vi "Write setSpectTempSetpoint.vi"(8 "error in (no error)":errorcluster, 10 "command_setSpectTempSetpoint":T1, 11 "setSpectTempSetpoint in":refnum<class "setSpectTempSetpoint.lvclass">) -> (0 "error out":errorcluster, 3 "setSpectTempSetpoint out":refnum<class "setSpectTempSetpoint.lvclass">)   [LabVIEW 2016, in "Commands.lvlib" / "setSpectTempSetpoint.lvclass"]
uses:
  setSpectTempSetpoint.lvclass
  ts_sallv_sedspectrometer/DataTypes/command_setSpectTempSetpoint.ctl
  setSpectTempSetpoint.lvclass/setSpectTempSetpoint.ctl
  ts_sallv_sedspectrometer/SALLV_sedSpectrometer.lvlib
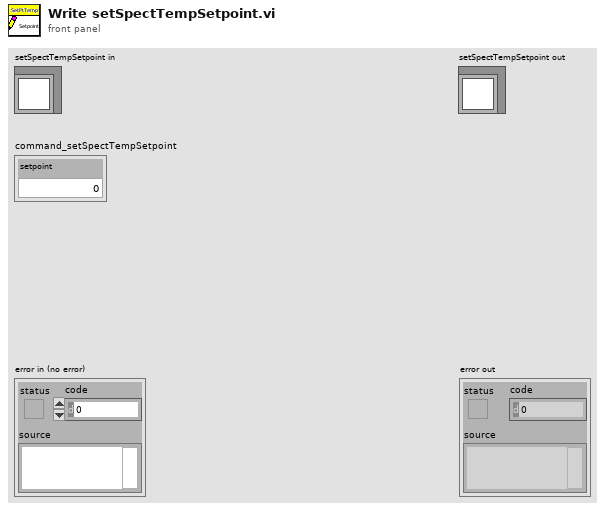
[diagram p1: front panel]
types:
  T1 = typedef "SALLV_sedSpectrometer.lvlib/command_setSpectTempSetpoint.ctl" = cluster{"setpoint":sgl}
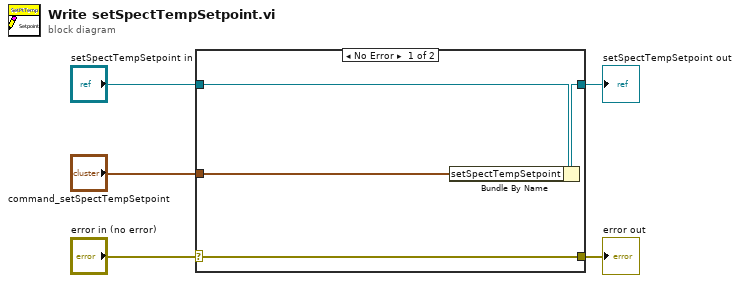
[diagram p0: block diagram]
diagram:
  n1 = case shown="No Error" "error in (no error)" {
    selector: "error in (no error)" -> [w9 w10]
    tunnel: [w9 w10] -> w4
    tunnel: [w7 w11] -> w2
    tunnel: "setSpectTempSetpoint in" -> [w8 w11]
    tunnel: "command_setSpectTempSetpoint" -> [w6 _]
    frame No Error {
      n2 = Bundle By Name(cluster=w8, "setSpectTempSetpoint"=w6) -> (w7:refnum<class "setSpectTempSetpoint.lvclass">)
    }
    frame Error {
    }
  }
  "error out" <- w4
  "setSpectTempSetpoint out" <- w2
